vi "Agilent_Init.vi"(2 "error in (no error)":errorcluster, 3 "Voltage Limit":dbl, 4 "Voltage Protection":dbl, 5 "VISA name":refnum<visa-resource-name>="TCPIP0::192.168.0.102::inst0::INSTR") -> (0 "error out":errorcluster, 1 "VISA resource name":refnum<visa-resource-name>)   [LabVIEW 2017]
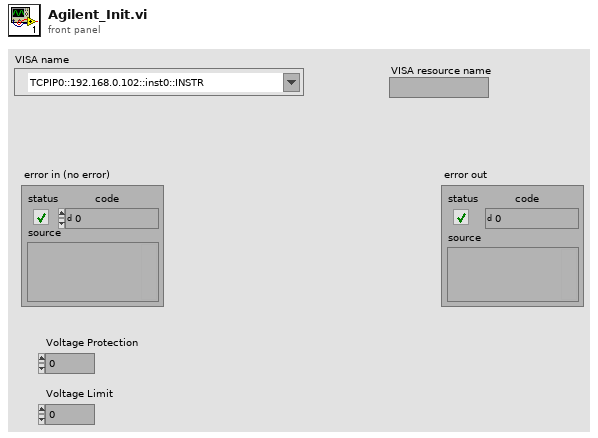
[diagram p1: front panel]
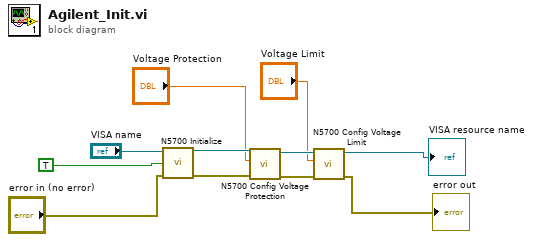
[diagram p0: block diagram]
diagram:
  n1 = call <instrlib>:"N5700 Initialize.vi"("VISA name"="VISA name", "Reset (T)"=TRUE, "error in (no error)"="error in (no error)") -> ("VISA out"=w10:refnum<visa-resource-name>, "error out"=w11:errorcluster)  [unwired: 11 in]
  n2 = call <instrlib>:"N5700 Config Voltage Protection.vi"("error"=w11, "OVP Level"="Voltage Protection", "VISA"=w10) -> ("error out"=w8:errorcluster, "VISA out"=w9:refnum<visa-resource-name>)  [unwired: 4 in]
  n3 = call <instrlib>:"N5700 Config Voltage Limit.vi"("error"=w8, "Volt Limit"="Voltage Limit", "VISA"=w9) -> ("error out"=→"error out":errorcluster, "VISA out"=→"VISA resource name":refnum<visa-resource-name>)  [unwired: 4 in]
